vi "Zero Power Meter.vi"(8 "error in (no error)":errorcluster, 11 "EXFO in":refnum<class "EXFO.lvclass">) -> (0 "error out":errorcluster, 3 "EXFO out":refnum<class "EXFO.lvclass">)   [LabVIEW 2018, in "EXFO.lvlib" / "EXFO.lvclass"]
doc: "This is a parent VI, the child VI will overwrite the functionality of this VI. \n\nThe purpose of the VI is to Tare/Zero the Power Meter. Programmatically, it must be confirmed that no input signal is injected into the system (or that the reference signal is input).\n\nAuthor: Ron Dexter\nCompany: Luminar\nModified: 5/20/2018"
uses:
  EXFO.lvclass
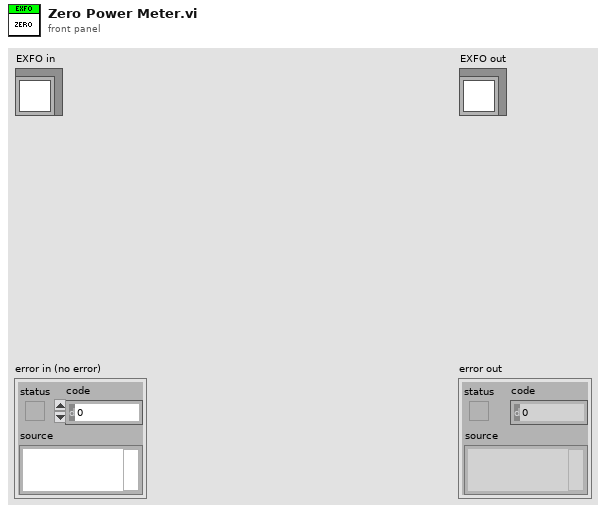
[diagram p1: front panel]
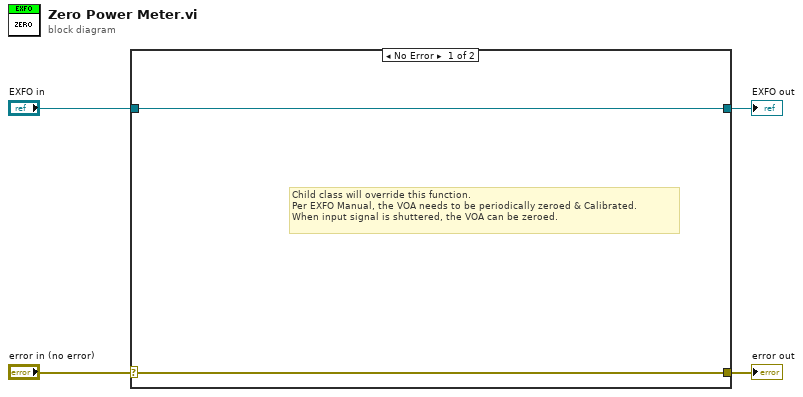
[diagram p0: block diagram]
diagram:
  n1 = case shown="No Error" "error in (no error)" {
    selector: "error in (no error)" -> [w5 w8]
    tunnel: [w5 w8] -> w3
    tunnel: [w6 w7] -> w1
    tunnel: "EXFO in" -> [w6 w7]
    frame No Error {
      # "Child class will override this function.\nPer EXFO Manual, the VOA needs to be periodically zeroed & Calibrated.  \nWhen input signal is shuttered, the VOA can be zeroed."
    }
    frame Error {
    }
  }
  "error out" <- w3
  "EXFO out" <- w1
